vi "Error Converter (ErrCode or Status).vi"(7 "error code":u32, 8 "return type":i32, 10 "error in (no error)":errorcluster) -> (3 "error out":errorcluster)   [LabVIEW 2017, in "maxonEPOS.lvlib"]
doc: "<B>VI</B> returns error code."
uses:
  Examples/maxonEPOS.lvlib
  Resources/EposCmd.dll
  SSI_Tool/InstrumentsInterfaces/Motordriver/maxon EPOS/Resources/EposCmd64.dll
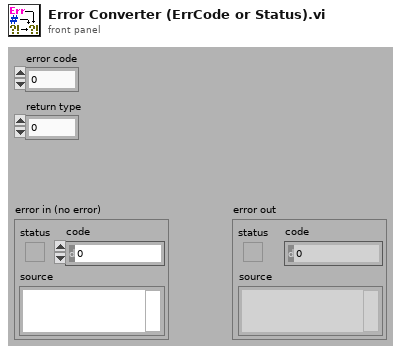
[diagram p1: front panel]
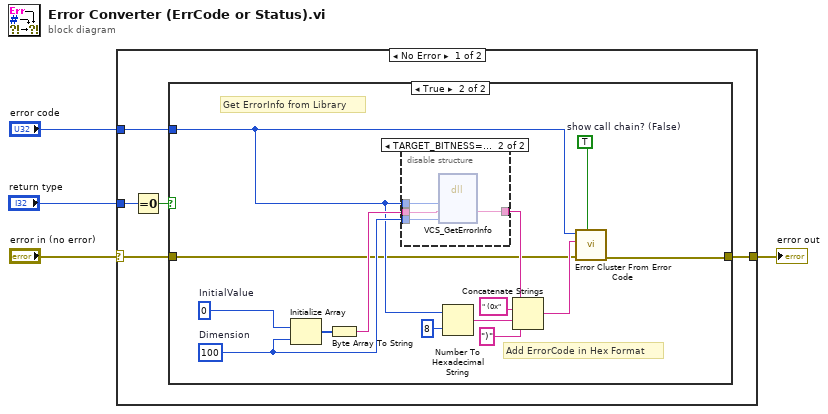
[diagram p0: block diagram]
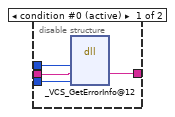
[diagram p3: hidden frame]
diagram:
  n1 = case shown="No Error" "error in (no error)" {
    selector: "error in (no error)" -> [w8 w33]
    tunnel: [w6 w33] -> w3
    tunnel: "error code" -> [w7 _]
    tunnel: "return type" -> [w5 _]
    frame No Error {
      n2 = Equal To 0?(x=w5) -> (x = 0?=w9:bool)
      n3 = case shown="True" w9 {
        tunnel: w8 -> [w10 w12]
        tunnel: w7 -> [_ w13]
        tunnel: [w10 w11] -> w6
        frame False {
        }
        frame True {
          w20 = 100  # Dimension
          w23 = 0  # InitialValue
          w24 = TRUE  # show call chain? (False)
          # "Add ErrorCode in Hex Format"
          # "Get ErrorInfo from Library"
          n4 = Initialize Array(w23, w20) -> (w22:i32[])
          n5 = Byte Array To String(unsigned byte array=w22) -> (string=w21:string)
          n6 = disable-structure shown="TARGET_BITNESS==64" {
            disable-tunnel: w21 -> [w28 w32]
            disable-tunnel: w20 -> [w27 w31]
            disable-tunnel: [w26 w30] -> w15
            disable-tunnel: w13 -> [w25 w29]
            frame condition #0 (active) {
              n7 = dll-call lib="C:/workspace/project/scancon/sw/SSI_Tool/InstrumentsInterfaces/Motordriver/maxon EPOS/Resources/EposCmd.dll" fn="_VCS_GetErrorInfo@12"("ErrorCodeValue"=w25, "ErrorInfo"=w28, "MaxStringSize"=w27) -> ("ErrorInfo"=w26:string)  [unwired: 6 in, 2 out]
            }
            frame condition #1 {
              n8 = dll-call lib="C:/Sources/LabView/maxon EPOS/Resources/EposCmd64.dll" fn="VCS_GetErrorInfo"("ErrorCodeValue"=w29, "ErrorInfo"=w32, "MaxStringSize"=w31) -> ("ErrorInfo"=w30:string)  [unwired: 6 in, 2 out]
            }
          }
          n9 = Number To Hexadecimal String(1:i16 8 ("width (-)"), 2:w13) -> (0:w18:string)
          n10 = Concatenate Strings(w15, " (0x" ("string"), w18, ")" ("string")) -> (w14:string)
          n11 = call <vilib>:"Error Cluster From Error Code.vi"("show call chain? (False)"=w24, "error in (no error)"=w12, "error message (\"\")"=w14, "error code (0)"=w13) -> ("error out"=w11:errorcluster)  [unwired: 5 in]
        }
      }
    }
    frame Error {
    }
  }
  "error out" <- w3
